vi "FindDefaultGateway.vi"() -> (2 "SubNet":string, 3 "Default Gateway":string)   [LabVIEW 2013]
uses:
  <vilib>/regexp/Match Regular Expression.xnode
panel:
  out "standard output":string
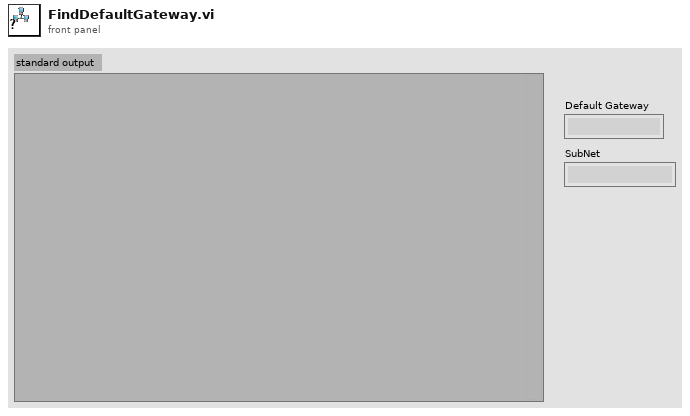
[diagram p1: front panel]
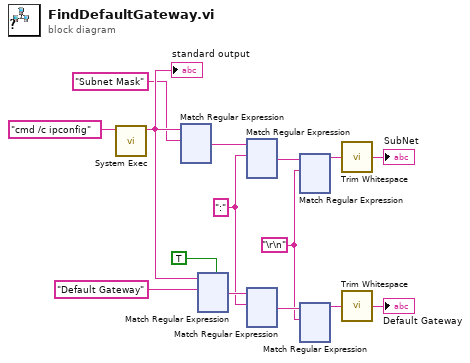
[diagram p0: block diagram]
diagram:
  w3 = "\r\n"
  w5 = ":" ("regular expression")
  n1 = call <vilib>:"System Exec.vi"("command line"="cmd /c ipconfig") -> ("standard output"=w8:string)  [unwired: 7 in, 3 out]
  "standard output" <- w8
  n2 = xnode "Match Regular Expression"("input string"=w8, "regular expression"="Subnet Mask") -> ("after match"=w6:string)  [unwired: 4 in, 4 out]
  n3 = xnode "Match Regular Expression"("input string"=w8, "regular expression"="Default Gateway" ("search string"), "multiline? (F)"=TRUE) -> ("after match"=w12:string)  [unwired: 3 in, 4 out]
  n4 = xnode "Match Regular Expression"("input string"=w6, "regular expression"=w5) -> ("after match"=w4:string)  [unwired: 4 in, 4 out]
  n5 = xnode "Match Regular Expression"("input string"=w12, "regular expression"=w5) -> ("after match"=w11:string)  [unwired: 4 in, 4 out]
  n6 = xnode "Match Regular Expression"("input string"=w4, "regular expression"=w3) -> ("before match"=w2:string)  [unwired: 4 in, 4 out]
  n7 = xnode "Match Regular Expression"("input string"=w11, "regular expression"=w3) -> ("before match"=w10:string)  [unwired: 4 in, 4 out]
  n8 = call <vilib>:"Trim Whitespace.vi"("string"=w2) -> ("trimmed string"=→"SubNet":string)  [unwired: 1 in]
  n9 = call <vilib>:"Trim Whitespace.vi"("string"=w10) -> ("trimmed string"=→"Default Gateway":string)  [unwired: 1 in]
